vi "ABB Report Noise.vi"(10 "Report in":string) -> (2 "Report out":string)   [LabVIEW 2017]
uses:
  ABB global.vi
panel:
  in  "Case Constant\n(See Context Help)":bool=TRUE
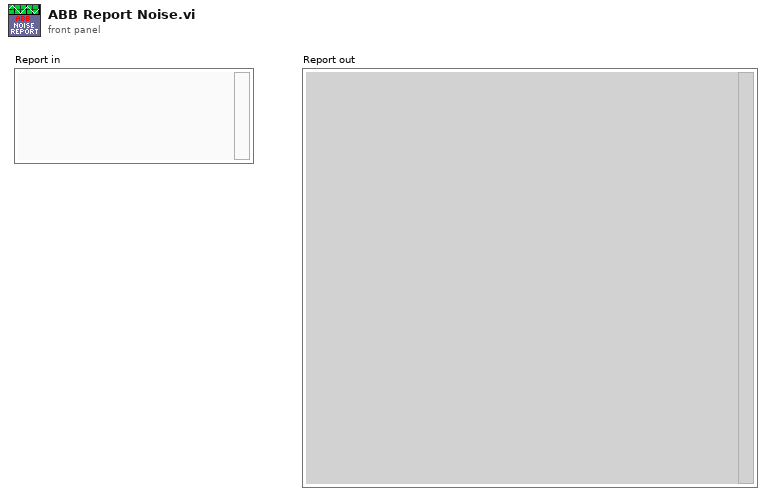
[diagram p1: front panel]
types:
  T1 = cluster{"Noise Before":string, "Noise During":string}
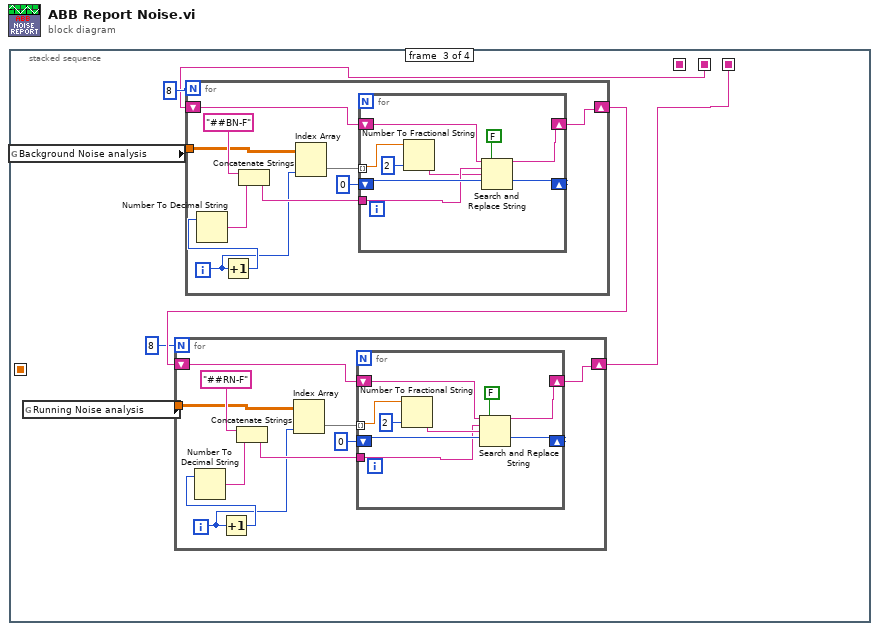
[diagram p0: block diagram]
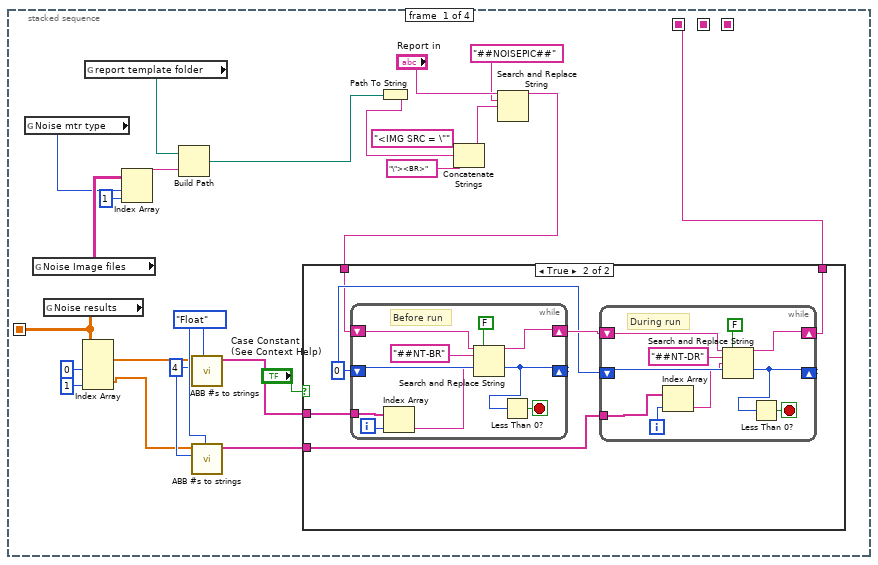
[diagram p2: hidden frame]
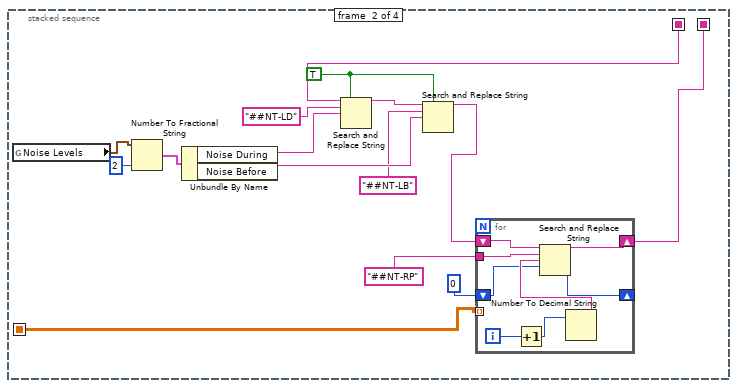
[diagram p4: hidden frame]
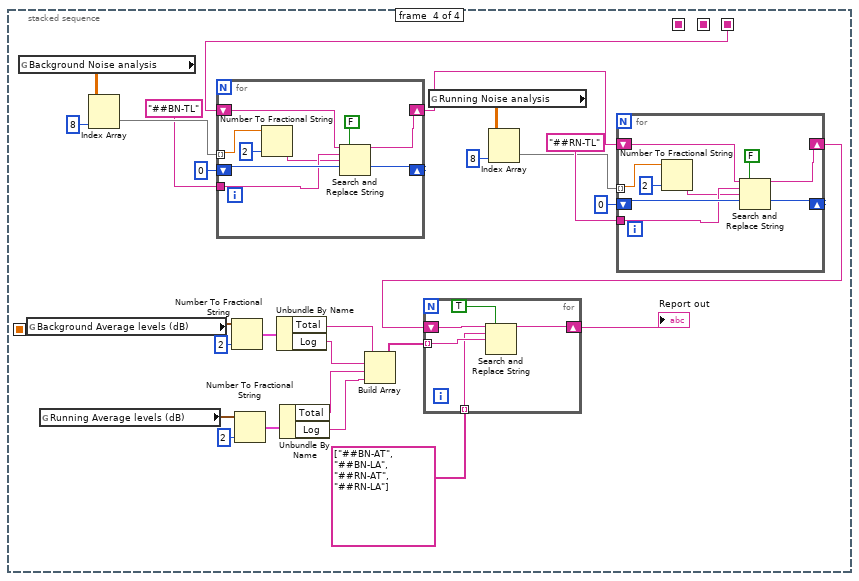
[diagram p5: hidden frame]
diagram:
  n1 = stacked-sequence {
    seq-local: [w8 _ _ _] -> [_ w66 _ _]
    seq-local: [w2 _ _ _] -> [_ w56 _ _]
    seq-local: [_ w52 _ _] -> [_ _ w79 _]
    seq-local: [_ _ w75 _] -> [_ _ _ w144]
    frame #0 {
      w11 = enum16{"Float", "Relative time HH:MM"}."Float" ("# type")
      w7 = 4 ("Precision")
      n2 = global read "ABB global.vi" "Noise mtr type"() -> (w1:i32)
      n3 = global read "ABB global.vi" "Noise Image files"() -> (w15:string[][])
      n4 = global read "ABB global.vi" "Noise results"() -> (w2:dbl[][])
      n5 = Index Array(array=w2, index (col) #1=0 ("disabled index (col)"), index (col) #2=1 ("index (col)")) -> (element #1=w6:dbl[], element #2=w5:dbl[])  [unwired: 2 in]
      n6 = global read "ABB global.vi" "report template folder"() -> (w18:path)
      n7 = Index Array(array=w15, index (row)=w1, index (col)=1 ("disabled index (col)")) -> (element=w16:string)
      n8 = Build Path(base path=w18, name or relative path=w16) -> (appended path=w17:path)
      n9 = call "ABB #s to strings.vi"("# type"=w11, "Precision"=w7, "Numbers in"=w6) -> ("Strings out"=w13:string[])  [unwired: 8 in]
      n10 = call "ABB #s to strings.vi"("# type"=w11, "Precision"=w7, "Numbers in"=w5) -> ("Strings out"=w12:string[])  [unwired: 8 in]
      n11 = Path To String(path=w17) -> (string=w21:string)
      n12 = Concatenate Strings("<IMG SRC = \"", w21, "\"><BR>" ("string")) -> (w22:string)
      n13 = Search and Replace String(input string="Report in", search string="##NOISEPIC##", replace string=w22) -> (result string=w9:string)  [unwired: 5 in, 3 out]
      n14 = case shown="True" "Case Constant\n(See Context Help)" {
        tunnel: w13 -> [_ w30]
        tunnel: w12 -> [_ w29]
        tunnel: w9 -> [w25 w27]
        tunnel: [w25 w26] -> w8
        frame False {
        }
        frame True {
          w28 = 0
          n15 = while {
            shift-right: [w49] -> w31
            shift-left: w27 -> [w51]
            tunnel: w30 -> [w44]
            shift-right: [w45] -> _
            shift-left: w28 -> [w48]
            i -> [w43]
            stop <- w46 stop-if-true
            # "Before run"
            n16 = Index Array(array=w44, index=w43) -> (element=w42:string)
            n17 = Search and Replace String(replace all?=FALSE ("replace all? (F)"), input string=w51, search string="##NT-BR", replace string=w42, offset=w48) -> (result string=w49:string, offset past replacement=w45:i32)  [unwired: 3 in, 2 out]
            n18 = Less Than 0?(x=w45) -> (x < 0?=w46:bool)
          }
          n19 = while {
            shift-right: [w39] -> w26
            shift-left: w31 -> [w41]
            tunnel: w29 -> [w34]
            shift-right: [w35] -> _
            shift-left: w28 -> [w38]
            i -> [w33]
            stop <- w36 stop-if-true
            # "During run"
            n20 = Index Array(array=w34, index=w33) -> (element=w32:string)
            n21 = Search and Replace String(replace all?=FALSE ("replace all? (F)"), input string=w41, search string="##NT-DR", replace string=w32, offset=w38) -> (result string=w39:string, offset past replacement=w35:i32)  [unwired: 3 in, 2 out]
            n22 = Less Than 0?(x=w35) -> (x < 0?=w36:bool)
          }
        }
      }
    }
    frame #1 {
      w57 = TRUE ("replace all? (F)")
      n23 = global read "ABB global.vi" "Noise Levels"() -> (w62:cluster{"Noise Before":dbl, "Noise During":dbl})
      n24 = Number To Fractional String(number=w62, precision (6)=i16 2) -> (F-format string=w63:T1)  [unwired: 2 in]
      n25 = Unbundle By Name(w63) -> ("Noise During"=w64:string, "Noise Before"=w59:string)
      n26 = Search and Replace String(replace all?=w57, input string=w66, search string="##NT-LD", replace string=w64) -> (result string=w60:string)  [unwired: 4 in, 3 out]
      n27 = Search and Replace String(replace all?=w57, input string=w60, search string="##NT-LB", replace string=w59) -> (result string=w53:string)  [unwired: 4 in, 3 out]
      n28 = for {
        tunnel: w56 -> [_] mode=indexing
        shift-right: [w69] -> _
        shift-left: 0 -> [w70]
        tunnel: "##NT-RP" ("search string") -> [w71]
        shift-right: [w68] -> w52
        shift-left: w53 -> [w67]
        i -> [w74]
        n29 = Increment(x=w74) -> (x+1=w73:i32)
        n30 = Number To Decimal String(number=w73) -> (decimal integer string=w72:string)  [unwired: 1 in]
        n31 = Search and Replace String(input string=w67, search string=w71, replace string=w72, offset=w70) -> (result string=w68:string, offset past replacement=w69:i32)  [unwired: 4 in, 2 out]
      }
    }
    frame #2 {
      n32 = global read "ABB global.vi" "Background Noise analysis"() -> (w80:dbl[][])
      n33 = global read "ABB global.vi" "Running Noise analysis"() -> (w77:dbl[][])
      n34 = for {
        N: 8 -> [_]
        tunnel: w80 -> [w107]
        shift-right: [w102] -> w78
        shift-left: w79 -> [w103]
        i -> [w101]
        n35 = Increment(x=w101) -> (x+1=w106:i32)
        n36 = Number To Decimal String(number=w106) -> (decimal integer string=w109:string)  [unwired: 1 in]
        n37 = Concatenate Strings("##BN-F", w109) -> (w108:string)
        n38 = Index Array(array=w107, index (col)=w101) -> (element=w105:dbl[])  [unwired: 1 in]
        n39 = for {
          shift-right: [w119] -> w102
          shift-left: w103 -> [w115]
          tunnel: w108 -> [w112]
          shift-right: [w116] -> _
          shift-left: 0 ("offset past replacement") -> [w118]
          tunnel: w105 -> [w114] mode=indexing
          n40 = Number To Fractional String(number=w114, precision (6)=i16 2) -> (F-format string=w111:string)  [unwired: 2 in]
          n41 = Search and Replace String(replace all?=FALSE ("replace all? (F)"), input string=w115, search string=w112, replace string=w111, offset=w118) -> (result string=w119:string, offset past replacement=w116:i32)  [unwired: 3 in, 2 out]
        }
      }
      n42 = for {
        N: 8 -> [_]
        tunnel: w77 -> [w88]
        shift-right: [w83] -> w75
        shift-left: w78 -> [w84]
        i -> [w82]
        n43 = Increment(x=w82) -> (x+1=w87:i32)
        n44 = Number To Decimal String(number=w87) -> (decimal integer string=w90:string)  [unwired: 1 in]
        n45 = Concatenate Strings("##RN-F", w90) -> (w89:string)
        n46 = Index Array(array=w88, index (col)=w82) -> (element=w86:dbl[])  [unwired: 1 in]
        n47 = for {
          shift-right: [w100] -> w83
          shift-left: w84 -> [w96]
          tunnel: w89 -> [w92]
          shift-right: [w97] -> _
          shift-left: 0 ("offset past replacement") -> [w99]
          tunnel: w86 -> [w95] mode=indexing
          n48 = Number To Fractional String(number=w95, precision (6)=i16 2) -> (F-format string=w93:string)  [unwired: 2 in]
          n49 = Search and Replace String(replace all?=FALSE ("replace all? (F)"), input string=w96, search string=w92, replace string=w93, offset=w99) -> (result string=w100:string, offset past replacement=w97:i32)  [unwired: 3 in, 2 out]
        }
      }
    }
    frame #3 {
      n50 = global read "ABB global.vi" "Background Noise analysis"() -> (w143:dbl[][])
      n51 = global read "ABB global.vi" "Background Average levels (dB)"() -> (w133:cluster{"Total":dbl, "Log":dbl})
      n52 = global read "ABB global.vi" "Running Average levels (dB)"() -> (w129:cluster{"Total":dbl, "Log":dbl})
      n53 = Index Array(array=w143, index (col)=8 ("disabled index (col)")) -> (element=w141:dbl[])  [unwired: 1 in]
      n54 = for {
        shift-right: [w168] -> w134
        shift-left: w144 -> [w164]
        tunnel: "##BN-TL" -> [w161]
        shift-right: [w165] -> _
        shift-left: 0 ("offset past replacement") -> [w167]
        tunnel: w141 -> [w163] mode=indexing
        n55 = Number To Fractional String(number=w163, precision (6)=i16 2) -> (F-format string=w160:string)  [unwired: 2 in]
        n56 = Search and Replace String(replace all?=FALSE ("replace all? (F)"), input string=w164, search string=w161, replace string=w160, offset=w167) -> (result string=w168:string, offset past replacement=w165:i32)  [unwired: 3 in, 2 out]
      }
      n57 = Number To Fractional String(number=w133, precision (6)=i16 2) -> (F-format string=w132:cluster{"Total":string, "Log":string})  [unwired: 2 in]
      n58 = Number To Fractional String(number=w129, precision (6)=i16 2) -> (F-format string=w128:cluster{"Total":string, "Log":string})  [unwired: 2 in]
      n59 = Unbundle By Name(w132) -> ("Total"=w126:string, "Log"=w125:string)
      n60 = Unbundle By Name(w128) -> ("Total"=w124:string, "Log"=w123:string)
      n61 = Build Array(w126, w125, w124, w123) -> (w122:string[])
      n62 = global read "ABB global.vi" "Running Noise analysis"() -> (w136:dbl[][])
      n63 = Index Array(array=w136, index (col)=8 ("disabled index (col)")) -> (element=w138:dbl[])  [unwired: 1 in]
      n64 = for {
        shift-right: [w159] -> w127
        shift-left: w134 -> [w155]
        tunnel: "##RN-TL" -> [w152]
        shift-right: [w156] -> _
        shift-left: 0 ("offset past replacement") -> [w158]
        tunnel: w138 -> [w154] mode=indexing
        n65 = Number To Fractional String(number=w154, precision (6)=i16 2) -> (F-format string=w151:string)  [unwired: 2 in]
        n66 = Search and Replace String(replace all?=FALSE ("replace all? (F)"), input string=w155, search string=w152, replace string=w151, offset=w158) -> (result string=w159:string, offset past replacement=w156:i32)  [unwired: 3 in, 2 out]
      }
      n67 = for {
        shift-right: [w149] -> w120
        shift-left: w127 -> [w150]
        tunnel: w122 -> [w148] mode=indexing
        tunnel: string[] ["##BN-AT", "##BN-LA", "##RN-AT", "##RN-LA"] -> [w147] mode=indexing
        n68 = Search and Replace String(replace all?=TRUE ("replace all? (F)"), input string=w150, search string=w147, replace string=w148) -> (result string=w149:string)  [unwired: 4 in, 3 out]
      }
      "Report out" <- w120
    }
  }
